vi "Test Label Drag.vi"(0 "FSM.Edge In":refnum<class "FSM.Edge.lvclass">, 9 "Coords":T1) -> (4 "FSM.Edge Out":refnum<class "FSM.Edge.lvclass">, 8 "drag label?":bool)   [LabVIEW 2020, in "FSM.Edge.lvclass"]
uses:
  FSM.Edge.lvclass
  <vilib>/Utility/miscctls.llb/LVPoint32TypeDef.ctl
  FSM.Edge.lvclass/FSM.Edge.ctl
  FSM.Label/FSM.Label.lvclass
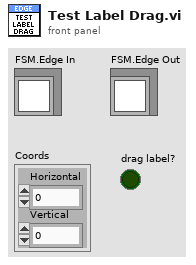
[diagram p1: front panel]
types:
  T1 = typedef "LVPoint32TypeDef.ctl" = cluster{"Horizontal":i32, "Vertical":i32}
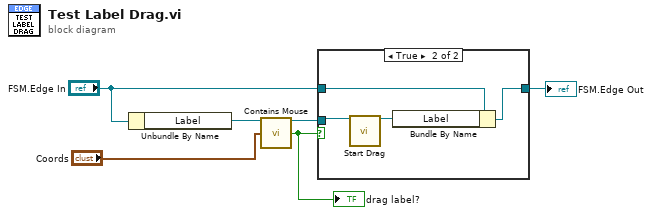
[diagram p0: block diagram]
diagram:
  n1 = Unbundle By Name("FSM.Edge In") -> ("Label"=w6:refnum<class "FSM.Label.lvclass">)
  n2 = call "Contains Mouse.vi"("FSM.Label"=w6, "Coords"="Coords") -> ("FSM.Label thru"=w3:refnum<class "FSM.Label.lvclass">, "contains mouse"=w4:bool)  [unwired: 12 in]
  "drag label?" <- w4
  n3 = case shown="True" w4 {
    tunnel: w3 -> [_ w11]
    tunnel: "FSM.Edge In" -> [w7 w10]
    tunnel: [w7 w8] -> w1
    frame False {
    }
    frame True {
      n4 = call "Start Drag.vi"("FSM.Label In"=w11) -> ("FSM.Label Out"=w9:refnum<class "FSM.Label.lvclass">)  [unwired: 14 in]
      n5 = Bundle By Name(cluster=w10, "Label"=w9) -> (w8:refnum<class "FSM.Edge.lvclass">)
    }
  }
  "FSM.Edge Out" <- w1
